vi "Configure Alarm Mark Com.vi"(0 "VISA resource name":refnum<visa-resource-name>, 1 "Color 1":cluster{"R":i32, "G":i32, "B":i32} {"B" min=0 max=255 step=1; "G" min=0 max=255 step=1; "R" min=0 max=255 step=1}, 2 "Color 3":cluster{"R":i32, "G":i32, "B":i32} {"B" min=0 max=255 step=1; "G" min=0 max=255 step=1; "R" min=0 max=255 step=1}, 5 "Comm Channel (001)":string="001", 7 "Mark Type (0 : Alarm)":i32(ring) items=["Alarm", "Fixed"], 9 "Enable Scale Board (False)":bool, 11 "error in (no error)":errorcluster, 12 "Color 2":cluster{"R":i32, "G":i32, "B":i32} {"B" min=0 max=255 step=1; "G" min=0 max=255 step=1; "R" min=0 max=255 step=1}, 13 "Color 4":cluster{"R":i32, "G":i32, "B":i32} {"B" min=0 max=255 step=1; "G" min=0 max=255 step=1; "R" min=0 max=255 step=1}) -> (4 "VISA resource name out":refnum<visa-resource-name>, 6 "Comm Channel":string, 15 "error out":errorcluster)   [LabVIEW 2020, in "Yokogawa GX Series.lvlib"]
doc: "Sets the alarm point mark of com channels.\n\nCommand: SAlmMarkCom"
uses:
  <instrlib>/Yokogawa GX Series/Yokogawa GX Series.lvlib
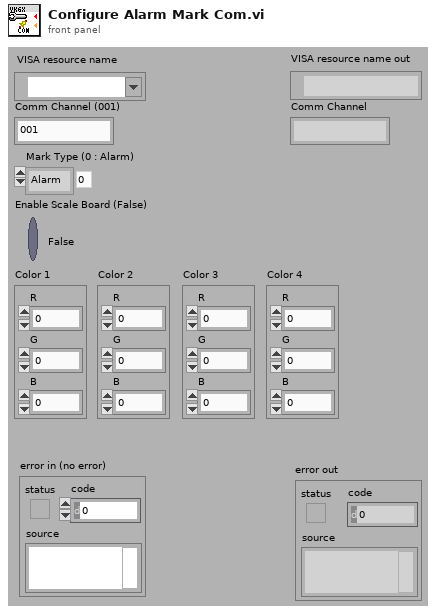
[diagram p1: front panel]
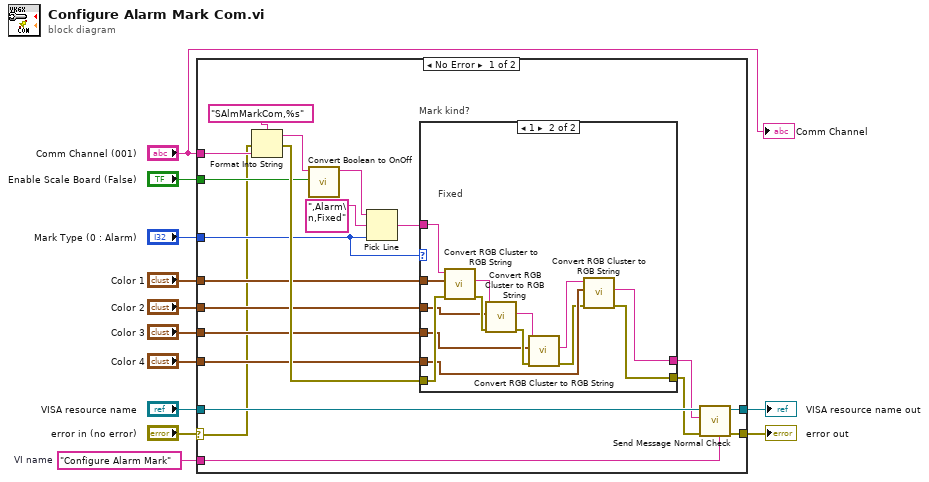
[diagram p0: block diagram]
diagram:
  w12 = "Configure Alarm Mark"  # VI name
  n1 = case shown="No Error" "error in (no error)" {
    selector: "error in (no error)" -> [w13 w49]
    tunnel: w12 -> [w31 _]
    tunnel: "VISA resource name" -> [w30 w50]
    tunnel: [w26 w50] -> w10
    tunnel: [w25 w49] -> w9
    tunnel: "Color 1" -> [w21 _]
    tunnel: "Color 2" -> [w20 _]
    tunnel: "Color 3" -> [w19 _]
    tunnel: "Color 4" -> [w18 _]
    tunnel: "Enable Scale Board (False)" -> [w16 _]
    tunnel: "Mark Type (0 : Alarm)" -> [w15 _]
    tunnel: "Comm Channel (001)" -> [w14 _]
    frame No Error {
      n2 = Format Into String(format string="SAlmMarkCom,%s", error in=w13, w14) -> (resulting string=w17:string, error out=w29:errorcluster)  [unwired: 1 in]
      n3 = call <instrlib>:"Convert Boolean to OnOff.vi"("On/Off"=w16, "Initial String (\"\")"=w17) -> ("Resulting String"=w23:string)  [unwired: 9 in]
      n4 = Pick Line(string ("")=w23, multi-line string=",Alarm\n,Fixed", line index=w15) -> (output string=w22:string)
      n5 = case "Mark kind?" shown="1" w15 {
        tunnel: [w33 w35] -> w27
        tunnel: [w34 w36] -> w28
        tunnel: w22 -> [w34 w40]
        tunnel: w29 -> [w33 w47]
        tunnel: w21 -> [_ w48]
        tunnel: w20 -> [_ w45]
        tunnel: w19 -> [_ w43]
        tunnel: w18 -> [_ w42]
        frame 0, Default {
          # "Alarm"
        }
        frame 1 {
          # "Fixed"
          n6 = call <instrlib>:"Convert RGB Cluster to RGB String.vi"("error in (no error)"=w47, "RGB"=w48, "Initial String"=w40) -> ("error out"=w46:errorcluster, "RGB String"=w39:string)  [unwired: 7 in]
          n7 = call <instrlib>:"Convert RGB Cluster to RGB String.vi"("error in (no error)"=w46, "RGB"=w45, "Initial String"=w39) -> ("error out"=w44:errorcluster, "RGB String"=w38:string)  [unwired: 7 in]
          n8 = call <instrlib>:"Convert RGB Cluster to RGB String.vi"("error in (no error)"=w44, "RGB"=w43, "Initial String"=w38) -> ("error out"=w41:errorcluster, "RGB String"=w37:string)  [unwired: 7 in]
          n9 = call <instrlib>:"Convert RGB Cluster to RGB String.vi"("error in (no error)"=w41, "RGB"=w42, "Initial String"=w37) -> ("error out"=w35:errorcluster, "RGB String"=w36:string)  [unwired: 7 in]
        }
      }
      n10 = call <instrlib>:"Send Message Normal Check.vi"("Source (\"\")"=w31, "error in (no error)"=w27, "Send Message (\"\")"=w28, "VISA resource name"=w30) -> ("error out"=w25:errorcluster, "VISA resource name out"=w26:refnum<visa-resource-name>)  [unwired: 2 in, 4 out]
    }
    frame Error {
    }
  }
  "error out" <- w9
  "VISA resource name out" <- w10
  "Comm Channel" <- "Comm Channel (001)"
